vi "BMon_Process.vi"(7 "PhaseDelay":dbl=-90.0 format="%#_13g", 11 "Empty Bore-BMon-Spec":dbl[](array[numeric])=array[63000 elements]) -> (3 "BMonOut":dbl[](array[numeric]))   [LabVIEW 2021]
uses:
  <vilib>/Analysis/4window.llb/windowTd.ctl
  MPS_global_variables.vi
  <vilib>/measure/maspectr.llb/FFT Spectrum (Mag-Phase) for 1 Chan.vi
  <vilib>/measure/NI_MAPro.lvlib
  <vilib>/Analysis/NI_AALPro.lvlib
  <vilib>/measure/NI_MABase.lvlib
panel:
  out "Waveform Graph":dbl[](graph)
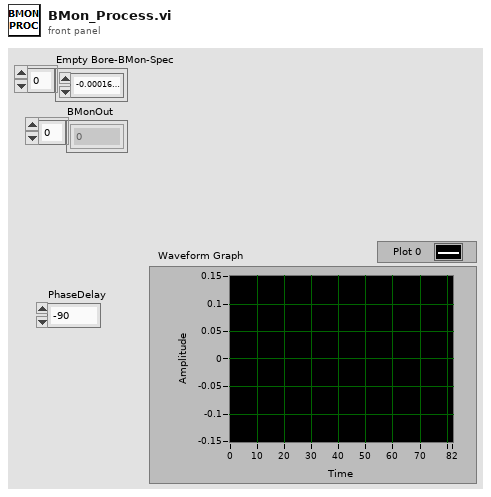
[diagram p1: front panel]
types:
  T1 = cluster{"sample rate":dbl, "Transmit frequency":dbl, "Transmit amplitude":dbl, "sample rate digital out":dbl, "TX cycles":i32, "sample rate DAQ1":dbl, "Receive frequency":dbl, "Receive range":dbl, "TX harmonics":dbl[]}
  T2 = typedef "NI_AALPro.lvlib/windowTd.ctl" = u32
  T3 = cluster{"sample rate":dbl, "Tx freq":dbl, "Tx amp":dbl, "Tx cycles\nSpectroscopy":dbl, "Bias amp":dbl, "Bias freq":dbl, "Receive range":dbl, "Bias Periods\nMagnetometry":dbl, "Tx Freq Division Factor":dbl, "Drive Periods per Bias":dbl, "TX harmonics":dbl[]}
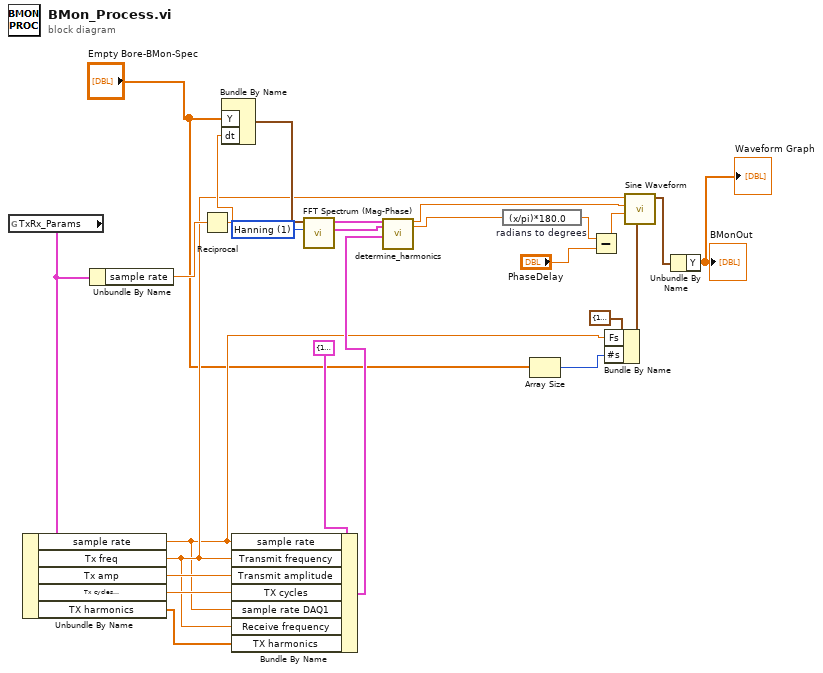
[diagram p0: block diagram]
diagram:
  w22 = T2 1 items=["Rectangle"=0, "Hanning"=1, "Hamming"=2, "Blackman-Harris"=3, "Exact Blackman"=4, "Blackman"=5, "Flat Top"=6, "4 Term B-Harris "=7, "7 Term B-Harris"=8, "Low Sidelobe"=9, "Blackman Nuttall"=11, "Triangle"=30, "Bartlett-Hanning"=31, "Bohman"=32, "Parzen"=33, "Welch"=34, "Kaiser"=60, "Dolph-Chebyshev"=61, "Gaussian"=62] ("window")
  n1 = global read "MPS_global_variables.vi" "TxRx_Params"() -> (w18:T3)
  n2 = Unbundle By Name(w18) -> ("sample rate"=w4:dbl, "Tx freq"=w11:dbl, "Tx amp"=w17:dbl, "Tx cycles\nSpectroscopy"=w16:dbl, "TX harmonics"=w15:dbl[])
  n3 = Unbundle By Name(w18) -> ("sample rate"=w25:dbl)
  n4 = Reciprocal(x=w25) -> (1/x=w24:dbl)
  n5 = Bundle By Name("Y"="Empty Bore-BMon-Spec", "dt"=w24) -> (w23:waveform(dbl))  [unwired: 1 in]
  n6 = Bundle By Name(cluster=T1 {"sample rate"=1000000.0, "Transmit frequency"=25000.0, "Transmit amplitude"=1.577, "sample rate digital out"=40000.0, "TX cycles"=600, "sample rate DAQ1"=1000000.0, "Receive frequency"=75000.0, "Receive range"=1.0, "TX harmonics"=[50000.0, 75000.0, 100000.0, 125000.0, 150000.0, 175000.0, 200000.0, 225000.0]} ("TxRxParams"), "sample rate"=w4, "Transmit frequency"=w11, "Transmit amplitude"=w17, "TX cycles"=w16, "sample rate DAQ1"=w4, "Receive frequency"=w11, "TX harmonics"=w15) -> (w14:T1)
  n7 = call-poly <vilib>:"FFT Spectrum (Mag-Phase).vi"("window"=w22, "time signal"=w23) -> ("phase"=w20:cluster{"f0":dbl, "df":dbl, "phase":dbl[]}, "magnitude"=w21:cluster{"f0":dbl, "df":dbl, "magnitude":dbl[]})  [unwired: 5 in, 3 out]
  n8 = call "determine_harmonics.vi"("FFT magnitude"=w21, "FFT phase"=w20, "TxRxParams"=w14) -> ("RX magnitude"=w12:dbl, "RX phase"=w13:dbl)  [unwired: 10 in, 5 out]
  n9 = expression code="(x/pi)*180.0" "radians to degrees"(w13) -> (w10:dbl)
  n10 = Array Size(array="Empty Bore-BMon-Spec") -> (size(s)=w2:i32)
  n11 = Subtract(x=w10, y="PhaseDelay") -> (x-y=w9:dbl)
  n12 = Bundle By Name(cluster=cluster{"Fs":dbl, "#s":dbl} {"Fs"=1000.0, "#s"=1000.0} ("sampling info"), "Fs"=w4, "#s"=w2) -> (w1:cluster{"Fs":dbl, "#s":dbl})
  n13 = call <vilib>:"Sine Waveform.vi"("sampling info"=w1, "phase"=w9, "amplitude"=w12, "frequency"=w11) -> ("signal out"=w7:waveform(dbl))  [unwired: 6 in, 1 out]
  n14 = Unbundle By Name(w7) -> ("Y"=→"BMonOut" →"Waveform Graph":dbl[])
